vi "Komponenten initialisieren.vi"(11 "Gasflasche":T3 items=["----"=10000, "IAG NH3 3000"=0, "IAG NH3 200"=1, "IAG NH3 2000"=2, "IAG MG"=3, "IAG O2"=4]) -> (2 "Komponente":T1, 3 "Sollwerte":T2)   [LabVIEW 2020, in "Erweiterte Konfig.lvlib" / "CG-Check Konfig.lvlib"]
uses:
  CG-Check Konfig.lvlib
  System Einstellungen V2/Gasflasche Auswahl.ctl
  System Einstellungen V2/Aktion FGV Gasbottledefinition.ctl
  FT-IR/FGV FT-IR Gasliste Aktionen.ctl
  <vilib>/regexp/Match Regular Expression.xnode
  System Einstellungen V2/System Einstellungen V2.lvlib
  FT-IR/FT-IR.lvlib
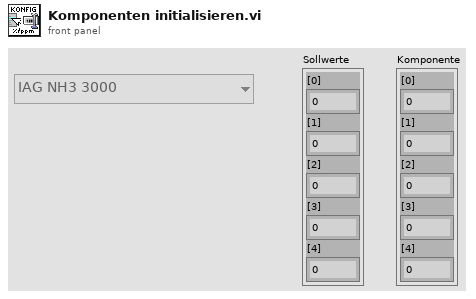
[diagram p1: front panel]
types:
  T1 = cluster{"[0]":i32, "[1]":i32, "[2]":i32, "[3]":i32, "[4]":i32}
  T2 = cluster{"[0]":dbl, "[1]":dbl, "[2]":dbl, "[3]":dbl, "[4]":dbl}
  T3 = typedef "System Einstellungen V2.lvlib/Gasflasche Auswahl.ctl" = u16
  T4 = typedef "System Einstellungen V2.lvlib/Aktion FGV Gasbottledefinition.ctl" = enum16{"lesen", "schreiben", "löschen", "laden", "speichern", "exportieren", "importieren"}
  T5 = typedef "System Einstellungen V2.lvlib/Gasflasche gesamt.ctl" = cluster{"Gasflasche":T6, "Trägergas":T7, "Komponenten":T8[]}
  T6 = typedef "System Einstellungen V2.lvlib/Gasflasche.ctl" = cluster{"Gasname für die Auswahl":string, "Chargennummer":string, "Ablaufdatum":timestamp}
  T7 = typedef "System Einstellungen V2.lvlib/Traegergas.ctl" = string
  T8 = typedef "System Einstellungen V2.lvlib/Gasflaschenkomponente.ctl" = cluster{"Gasauswahl":string, "Konzentration IST":dbl, "Einheit":string, "Genauigkeit":dbl}
  T9 = typedef "FT-IR.lvlib/FGV FT-IR Gasliste Aktionen.ctl" = enum16{"lesen", "Gasliste FT-IR", "Gasliste ausgelesen", "laden", "speichern", "löschen"}
  T10 = typedef "String - Ausgabefeld.ctl" = string
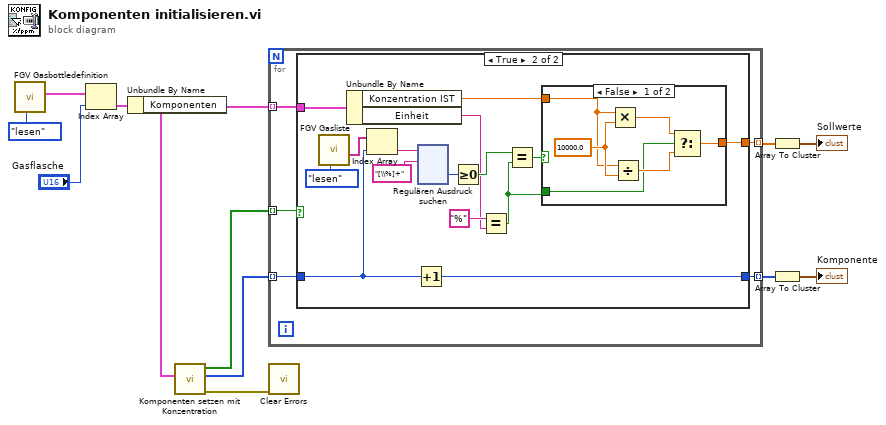
[diagram p0: block diagram]
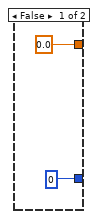
[diagram p2: hidden frame]
diagram:
  n1 = call "FGV Gasbottledefinition.vi"("Aktion"=Aktion_FGV_Gasbottledefinition."lesen") -> ("Gasflaschen Liste gesamt"=w8:T5[])  [unwired: 8 in, 2 out]
  n2 = Index Array(array=w8, index="Gasflasche") -> (element=w9:T5)
  n3 = Unbundle By Name(w9) -> ("Komponenten"=w10:T8[])
  n4 = call "Komponenten setzen mit Konzentration.vi"("Komponenten"=w10) -> ("error out"=w3:errorcluster, "Index"=w12:i32[], "found"=w11:bool[])  [unwired: 6 in, 2 out]
  n5 = for {
    tunnel: w11 -> [w17] mode=indexing
    tunnel: w12 -> [w16] mode=indexing
    tunnel: w10 -> [w15] mode=indexing
    tunnel: [w14] -> w6 mode=indexing
    tunnel: [w13] -> w5 mode=indexing
    n6 = case shown="True" w17 {
      tunnel: w16 -> [_ w20]
      tunnel: w15 -> [_ w34]
      tunnel: [0 w21] -> w14
      tunnel: [0.0 ("Konzentration IST ppm") w26] -> w13
      frame False {
      }
      frame True {
        n7 = call "FGV Gasliste.vi"("Aktionen"=FGV_FT-IR_Gasliste_Aktionen."lesen") -> ("Aktuelle Gasliste gesamt"=w22:T10[])  [unwired: 8 in, 2 out]
        n8 = Unbundle By Name(w34) -> ("Konzentration IST"=w27:dbl, "Einheit"=w25:string)
        n9 = Index Array(array=w22, index=w20) -> (element=w24:T10)
        n10 = Increment(x=w20) -> (x+1=w21:i32)
        n11 = xnode "Regulären Ausdruck suchen"("Eingangs-String"=w24, "Regulärer Ausdruck"="[\\%]+") -> ("Offset nach Übereinstimmung"=w33:i32)  [unwired: 4 in, 4 out]
        n12 = Greater Or Equal To 0?(x=w33) -> (x >= 0?=w28:bool)
        n13 = Equal?(x="%", y=w25) -> (x = y?=w29:bool)
        n14 = Equal?(x=w28, y=w29) -> (x = y?=w30:bool)
        n15 = case shown="False" w30 {
          tunnel: w27 -> [w38 w41]
          tunnel: [w36 w41] -> w26
          tunnel: w29 -> [w35 _]
          frame False {
            w39 = 10000.0 ("t")
            n16 = Multiply(x=w38, y=w39) -> (x*y=w40:dbl)
            n17 = Divide(x=w38, y=w39) -> (x/y=w37:dbl)
            n18 = Select(t=w40, s=w35, f=w37) -> (s? t:f=w36:dbl)
          }
          frame True {
          }
        }
      }
    }
  }
  n19 = call <vilib>:"Clear Errors.vi"("error in (no error)"=w3) -> ()  [unwired: 5 in, 2 out]
  n20 = Array To Cluster(array=w5) -> (cluster=→"Sollwerte":T2)
  n21 = Array To Cluster(array=w6) -> (cluster=→"Komponente":T1)
